vi "Fixturring.vi"(0 "Image CRL":T1(plugin-control), 5 "Main In":T2, 9 "Referance Listbox":string[](array[string]), 11 "error in":errorcluster) -> (2 "Angle":sgl, 3 "x = y?":bool, 4 "Fixturing?":bool, 6 "Fixturing ROI":i32[](array[numeric]), 8 "Main":T2, 10 "Image":T1(plugin-control), 13 "Score":sgl, 15 "error out":errorcluster)   [LabVIEW 2020]
uses:
  <vilib>/vision/Image Controls.llb/IMAQ Image.ctl
  <vilib>/vision/NI_Vision_Development_Module.lvlib
panel:
  out "Bounding Box":cluster{"x":sgl, "y":sgl}[](array[cluster])
  out "Number of Matches":i32
  out "Matches (real-world)":T3(array[cluster]) {"Bounding Box"."y" format="%.2f"; "Bounding Box"."x" format="%.2f"; "Score" format="%.2f"; "Scale" format="%.2f"; "Angle" format="%.2f"; "Position"."y" format="%.2f"; "Position"."x" format="%.2f"}
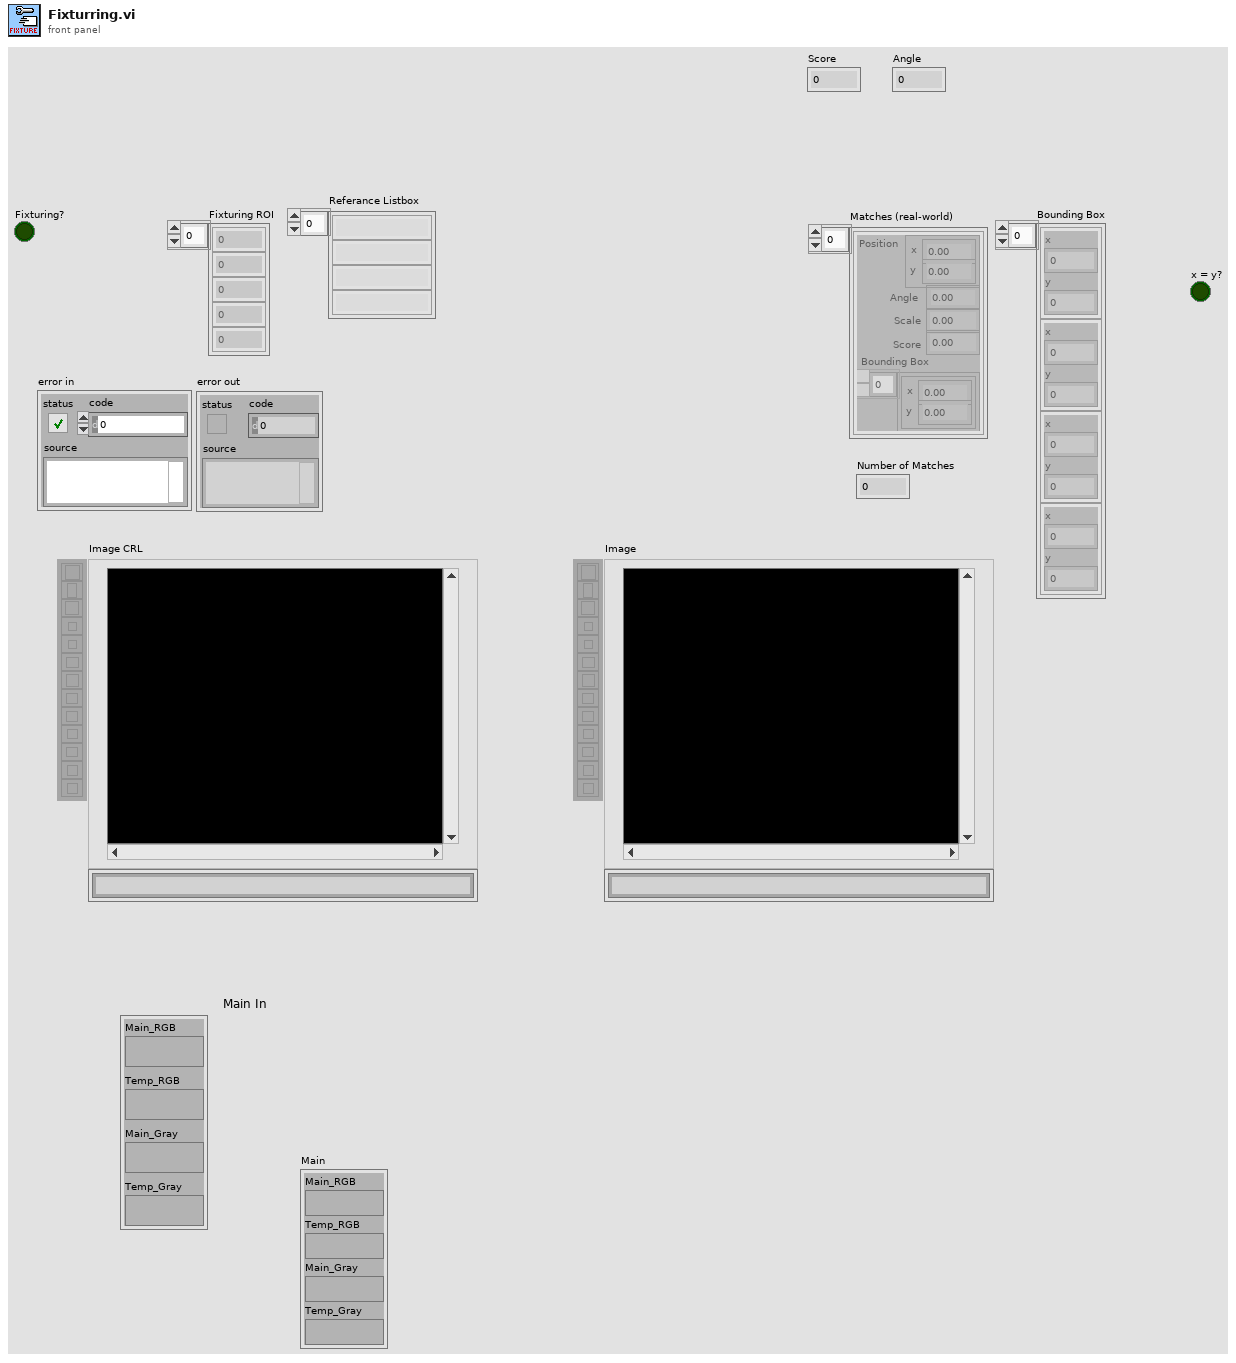
[diagram p1: front panel]
types:
  T1 = typedef "IMAQ Image.ctl" = refnum<image>
  T2 = cluster{"Main_RGB":T1, "Temp_RGB":T1, "Main_Gray":T1, "Temp_Gray":T1}
  T3 = cluster{"Position":cluster{"x":sgl, "y":sgl}, "Angle":sgl, "Scale":sgl, "Score":sgl, "Bounding Box":cluster{"x":sgl, "y":sgl}[]}[]
  T4 = cluster{"Global Rectangle":i32[], "Contours":cluster{"Contour Type":u32, "ROI Type":u32, "Points":i32[]}[]}
  T5 = cluster{"Number of Matches Requested":i32, "Minimum Match Score":sgl, "Angle Ranges":cluster{"Start Angle":sgl, "End Angle":sgl}[]}
  T6 = cluster{"Position":cluster{"x":sgl, "y":sgl}, "Angle":sgl, "Scale":sgl, "Score":sgl, "Bounding Box":cluster{"x":sgl, "y":sgl}[]}
  T7 = cluster{"Global Rectangle[0]":i32, "Global Rectangle[1]":i32, "Global Rectangle[2]":i32, "Global Rectangle[3]":i32}
  T8 = cluster{i32[], cluster{"Contour Type":u32, "Contour Type":i32, i32[]}[]}
  T9 = cluster{i32[], cluster{"Contour Type":u32, u32, i32[]}[]}
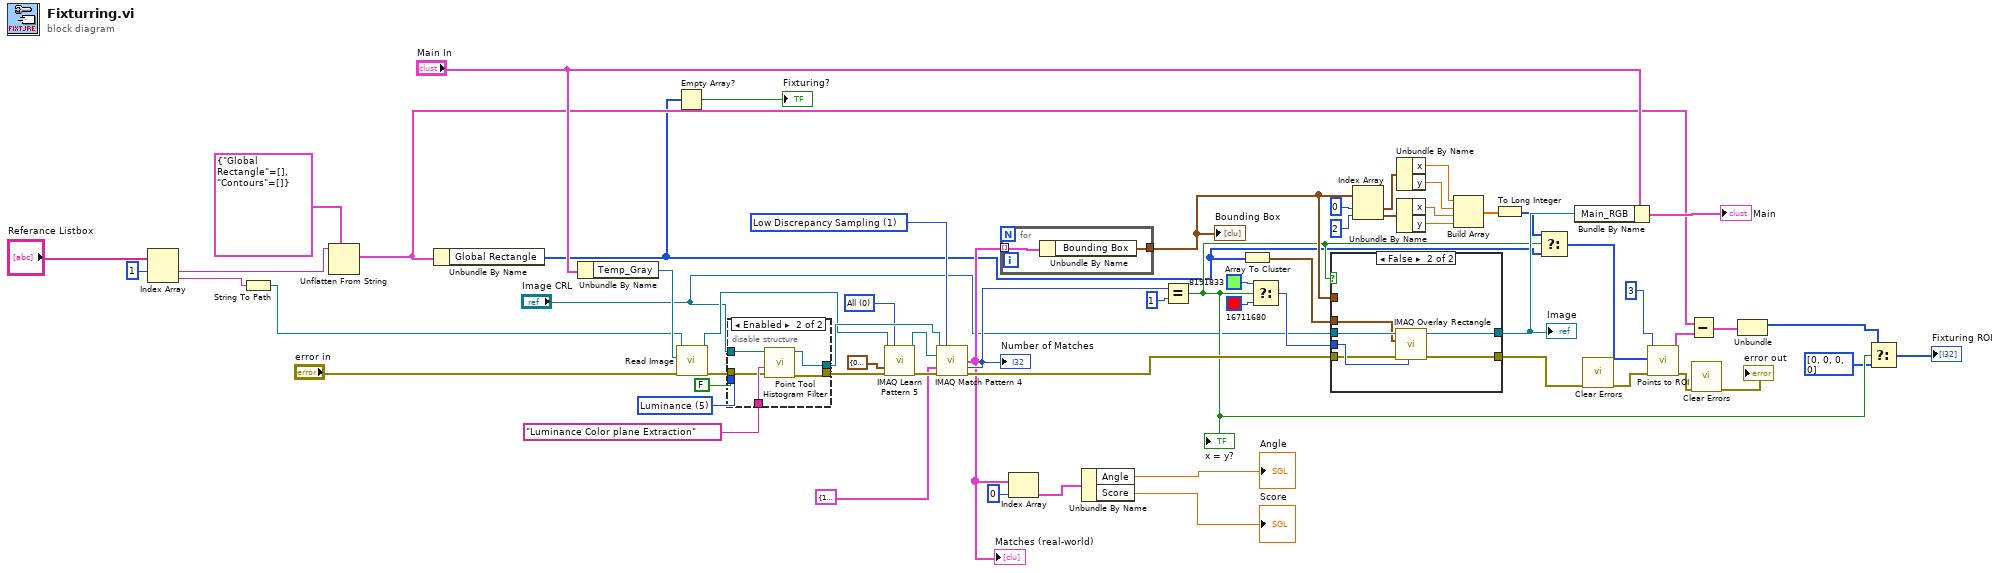
[diagram p0: block diagram]
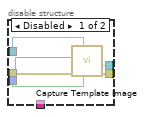
[diagram p2: hidden frame]
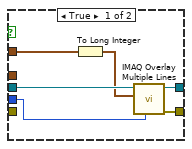
[diagram p3: hidden frame]
diagram:
  w23 = 0 items=["All", "Low Discrepancy Sampling", "Grayscale Value Pyramid", "Gradients Pyramid"] ("Algorithm")
  w29 = 5 items=["Red", "Green", "Blue", "Hue", "Saturation", "Luminance", "Value", "Intensity"] ("Color Plane")
  w55 = 1 items=["All", "Low Discrepancy Sampling", "Grayscale Value Pyramid", "Gradients Pyramid"] ("Algorithm")
  n1 = Index Array(array="Referance Listbox", index #1=1 ("index")) -> (element #1=w7:string, element #2=w4:string)  [unwired: 1 in]
  n2 = String To Path(string=w4) -> (path=w3:path)
  n3 = Unflatten From String(type=T4 {"Global Rectangle"=[], "Contours"=[]} ("ROI"), binary string=w7) -> (value=w6:T4)  [unwired: 3 in, 2 out]
  n4 = Unbundle By Name(w6) -> ("Global Rectangle"=w5:i32[])
  n5 = Unbundle By Name("Main In") -> ("Temp_Gray"=w57:T1)
  n6 = Empty Array?(array=w5) -> (empty?=→"Fixturing?":bool)
  n7 = call "Read Image.vi"("error in (no error)"="error in", "Image"=w57, "Image Path"=w3) -> ("error out"=w58:errorcluster, "Refnum out"=w24:T1)  [unwired: 7 in]
  n8 = disable-structure shown="Enabled" {
    disable-tunnel: [w69 w71] -> w61
    disable-tunnel: w58 -> [w68 w72]
    disable-tunnel: [w67 w70] -> w54
    disable-tunnel: FALSE ("RGB?Color") -> [w66 _]
    disable-tunnel: w29 -> [w65 _]
    disable-tunnel: "Image CRL" -> [w64 w74]
    disable-tunnel: "Luminance Color plane Extraction" ("Combo Box") -> [_ w73]
    frame Disabled {
      n9 = call "Capture Template Image.vi"("RGB?Color"=w66, "Main_RGB"=w64, "error in"=w68, "Color Plane"=w65) -> ("error out"=w69:errorcluster, "Main_Gray Out"=w67:T1)  [unwired: 6 in]
    }
    frame Enabled {
      n10 = call "Point Tool Histogram Filter.vi"("error in"=w72, "Combo Box"=w73, "Image in"=w74) -> ("error out"=w71:errorcluster, "Image out"=w70:T1)  [unwired: 7 in]
    }
  }
  n11 = call "IMAQ Learn Pattern 5"("Image"=w24, "Algorithm"=w23, "Angle Range"=cluster{"Start Angle":sgl, "End Angle":sgl} {"Start Angle"=0.0, "End Angle"=360.0}, "error in (no error)"=w61) -> ("Template Image Out"=w59:T1, "error out"=w60:errorcluster)  [unwired: 9 in, 1 out]
  n12 = call "IMAQ Match Pattern 4"("Image"=w54, "Algorithm"=w55, "Template Image"=w59, "Parameters"=T5 {"Number of Matches Requested"=1, "Minimum Match Score"=800.0, "Angle Ranges"=[{"Start Angle"=-100.0, "End Angle"=100.0}]}, "error in (no error)"=w60) -> ("Matches (real-world)"=w16:T3, "Number of Matches"=w53:i32, "error out"=w33:errorcluster)  [unwired: 6 in, 2 out]
  "Matches (real-world)" <- w16
  "Number of Matches" <- w53
  n13 = for {
    tunnel: w16 -> [w76] mode=indexing
    tunnel: [w75] -> w34
    n14 = Unbundle By Name(w76) -> ("Bounding Box"=w75:cluster{"x":sgl, "y":sgl}[])
  }
  "Bounding Box" <- w34
  n15 = Index Array(array=w16, index=0) -> (element=w14:T6)
  n16 = Unbundle By Name(w14) -> ("Angle"=→"Angle":sgl, "Score"=→"Score":sgl)
  n17 = Equal?(x=w53, y=1) -> (x = y?=w21:bool)
  "x = y?" <- w21
  n18 = Array To Cluster(array=w5) -> (cluster=w32:T7)
  n19 = Select(t=u32 8191833, s=w21, f=u32 16711680) -> (s? t:f=w49:u32)
  n20 = case shown="False" w21 {
    tunnel: "Image CRL" -> [w82 w87]
    tunnel: [w81 w86] -> w25
    tunnel: w49 -> [w79 w85]
    tunnel: [w78 w88] -> w37
    tunnel: w34 -> [w77 _]
    tunnel: w33 -> [_ w84]
    tunnel: w32 -> [_ w83]
    frame True {
      n21 = To Long Integer(number=w77) -> (32bit integer=w80:cluster{"x":i32, "y":i32}[])
      n22 = call "IMAQ Overlay Multiple Lines"("Color"=w79, "Line End Points"=w80, "Image"=w82) -> ("error out"=w78:errorcluster, "Image Out"=w81:T1)  [unwired: 3 in, 4 out]
    }
    frame False {
      n23 = call "IMAQ Overlay Rectangle"("Color"=w85, "error in (no error)"=w84, "Rectangle"=w83, "Image"=w87) -> ("error out"=w88:errorcluster, "Image Out"=w86:T1)  [unwired: 6 in]
    }
  }
  "Image" <- w25
  n24 = Index Array(array=w34, index #1=0 ("index"), index #2=2 ("index")) -> (element #1=w46:cluster{"x":sgl, "y":sgl}, element #2=w45:cluster{"x":sgl, "y":sgl})
  n25 = Unbundle By Name(w46) -> ("x"=w44:sgl, "y"=w43:sgl)
  n26 = Unbundle By Name(w45) -> ("x"=w42:sgl, "y"=w41:sgl)
  n27 = Build Array(w44, w43, w42, w41) -> (w39:sgl[])
  n28 = To Long Integer(number=w39) -> (32bit integer=w22:i32[])
  n29 = Select(t=w22, s=w21, f=w5) -> (s? t:f=w36:i32[])
  n30 = Bundle By Name(cluster="Main In", "Main_RGB"=w25) -> (→"Main":T2)
  n31 = call <vilib>:"Clear Errors.vi"("error in (no error)"=w37) -> ("error out"=w35:errorcluster)  [unwired: 5 in, 1 out]
  n32 = call "Points to ROI.vi"("error in (no error)"=w35, "Point_array"=w36, "Contour Type"=3) -> ("error out"=w28:errorcluster, "ROI"=w38:T8)  [unwired: 7 in]
  n33 = Subtract(x=w6, y=w38) -> (x-y=w63:T9)
  n34 = call <vilib>:"Clear Errors.vi"("error in (no error)"=w28) -> ("error out"=→"error out":errorcluster)  [unwired: 5 in, 1 out]
  n35 = Unbundle(w63) -> (w20:i32[])  [unwired: 1 out]
  n36 = Select(t=w20, s=w21, f=i32[] [0, 0, 0, 0]) -> (s? t:f=→"Fixturing ROI":i32[])
